vi "Set_Axis or coord System Name.vi"(8 "error in (no error)":errorcluster, 10 "Axis or coord System Name":string, 11 "MotionModule runtime_in":refnum<class "MotionModule runtime.lvclass">) -> (0 "error out":errorcluster, 3 "MotionModule runtime_out":refnum<class "MotionModule runtime.lvclass">)   [LabVIEW 2017, in "MotionModule runtime.lvclass"]
uses:
  MotionModule runtime.lvclass
  MotionModule runtime.lvclass/MotionModule runtime.ctl
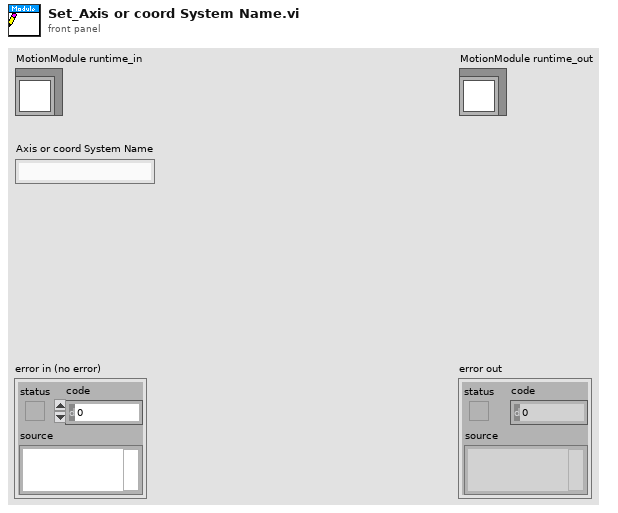
[diagram p1: front panel]
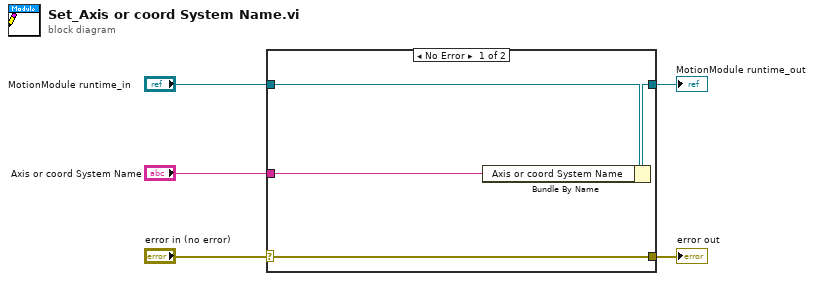
[diagram p0: block diagram]
diagram:
  n1 = case shown="No Error" "error in (no error)" {
    selector: "error in (no error)" -> [w9 w10]
    tunnel: [w9 w10] -> w4
    tunnel: [w7 w11] -> w2
    tunnel: "MotionModule runtime_in" -> [w8 w11]
    tunnel: "Axis or coord System Name" -> [w6 _]
    frame No Error {
      n2 = Bundle By Name(cluster=w8, "Axis or coord System Name"=w6) -> (w7:refnum<class "MotionModule runtime.lvclass">)
    }
    frame Error {
    }
  }
  "error out" <- w4
  "MotionModule runtime_out" <- w2
